vi "volt to level.vi"(1 "voltage /V":dbl) -> (0 "level":i16)   [LabVIEW 2017]
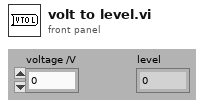
[diagram p1: front panel]
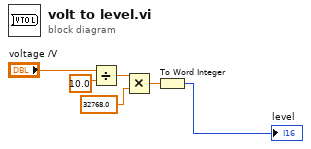
[diagram p0: block diagram]
diagram:
  n1 = Divide(x="voltage /V", y=10.0) -> (x/y=w3:dbl)
  n2 = Multiply(x=w3, y=32768.0) -> (x*y=w5:dbl)
  n3 = To Word Integer(number=w5) -> (16bit integer=→"level":i16)
